vi "StartWalkabout.vi"(0 "reference in":refnum<class "Object.lvclass">, 3 "ms timeout (-1)":i32=-1, 5 "error in (no error)":errorcluster) -> (14 "reference out":refnum<class "Object.lvclass">, 19 "error out":errorcluster)   [LabVIEW 2019, in "Object.lvclass"]
doc: "Looks up an existing object matching object name or creates a new object and returns a refnum you can use when calling other class methods.\n\nObjects created with this VI should be destroyed using this class Delete VI."
uses:
  Object.lvclass
panel:
  out "timed out":bool
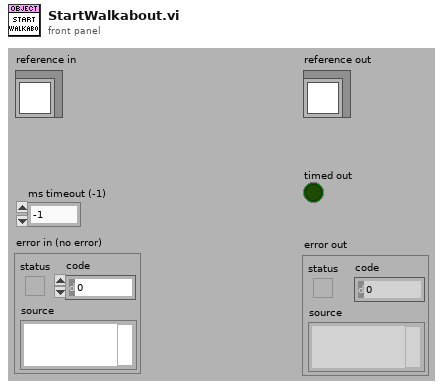
[diagram p1: front panel]
types:
  T1 = enum16{"ReadRepository", "CreateNew", "CreateOrLookUpExisting"}
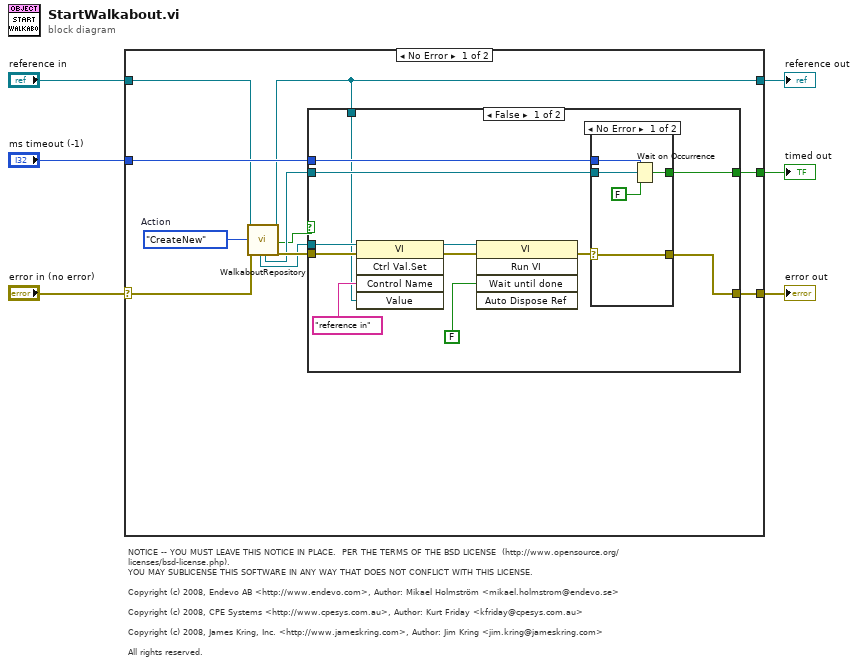
[diagram p0: block diagram]
diagram:
  # "NOTICE -- YOU MUST LEAVE THIS NOTICE IN PLACE.  PER THE TERMS OF THE BSD LICENSE  (http://www.opensource.org/licenses/bsd-license.php).\nYOU MAY SUBLICENSE THIS SOFTWARE IN ANY WAY THAT DOES NOT CONFLICT WITH THIS LICENSE.\n\nCopyright (c) 2008, Endevo AB <http://www.endevo.com>, Author: Mikael Holmström <mikael.holmstrom@endevo.se>\n\nCopyright (c) 2008, CPE Systems <http://www.cpesys.com.au>, Author: Kurt Friday <kfriday@cpesys.com.au>\n\nCopyright (c) 2008, James Kring, Inc. <http://www.jameskring.com>, Author: Jim Kring <jim.kring@jameskring.com>\n\nAll rights reserved."
  n1 = case shown="No Error" "error in (no error)" {
    selector: "error in (no error)" -> [w13 w37]
    tunnel: [w15 w37] -> w5
    tunnel: [w9 w38] -> w3
    tunnel: "reference in" -> [w7 w38]
    tunnel: "ms timeout (-1)" -> [w17 _]
    tunnel: [w16 _] -> w1
    frame No Error {
      w14 = T1."CreateNew"  # Action
      n2 = call "WalkaboutRepository.vi"("reference in"=w7, "Action(ReadRepository)"=w14, "error in (no error)"=w13) -> ("ProcessViRef"=w11:refnum<vi>, "ProcessSyncOccurrence"=w10:refnum<k4>, "reference out"=w9:refnum<class "Object.lvclass">, "ProcessAlreadyStarted"=w8:bool, "error out"=w12:errorcluster)  [unwired: 12 out]
      n3 = case shown="False" w8 {
        tunnel: w17 -> [w25 _]
        tunnel: [w24 _] -> w16
        tunnel: [w22 w36] -> w15
        tunnel: w12 -> [w21 w36]
        tunnel: w11 -> [w20 _]
        tunnel: w10 -> [w19 _]
        tunnel: w9 -> [w18 _]
        frame False {
          n4 = invoke class="VI" method="Ctrl Val.Set"(reference=w20, error in=w21, "Control Name"="reference in", "Value"=w18) -> (reference out=w28:refnum<vi>, error out=w27:errorcluster)  [unwired: 1 in, 3 out]
          n5 = invoke class="VI" method="Run VI"(reference=w28, error in=w27, "Wait until done"=FALSE ("Wait Until Done")) -> (error out=w23:errorcluster)  [unwired: 2 in, 4 out]
          n6 = case shown="No Error" w23 {
            tunnel: w19 -> [w33 _]
            tunnel: w25 -> [w32 _]
            tunnel: [w31 _] -> w24
            selector: w23 -> [w30 w35]
            tunnel: [w30 w35] -> w22
            frame No Error {
              n7 = Wait on Occurrence(1:FALSE ("ignore previous (T)"), 2:w33, 3:w32) -> (0:w31:bool)
            }
            frame Error {
            }
          }
        }
        frame True {
          # "Process Already started.\nThis option will only be used togeather with the\naction: \"CreateOrLookUpExisting\""
        }
      }
    }
    frame Error {
    }
  }
  "error out" <- w5
  "reference out" <- w3
  "timed out" <- w1
